vi "A x B (Optimized).vi"   [LabVIEW 2017, in "NI_AALBase.lvlib"]
uses:
  <vilib>/Analysis/NI_AALBase.lvlib
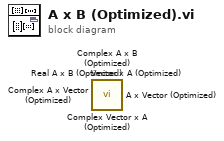
[diagram p0: block diagram]
diagram:
  n1 = call <vilib>:"Complex Vector x A (Optimized).vi"() -> ()  [unwired: 2 in, 2 out]
  n2 = call <vilib>:"Vector x A (Optimized).vi"() -> ()  [unwired: 2 in, 2 out]
  n3 = call <vilib>:"Complex A x Vector (Optimized).vi"() -> ()  [unwired: 2 in, 2 out]
  n4 = call <vilib>:"A x Vector (Optimized).vi"() -> ()  [unwired: 2 in, 2 out]
  n5 = call <vilib>:"Complex A x B (Optimized).vi"() -> ()  [unwired: 2 in, 2 out]
  n6 = call <vilib>:"Real A x B (Optimized).vi"() -> ()  [unwired: 2 in, 2 out]
